vi "Get Indicator Number.vi"(8 "error in (no error)":errorcluster, 11 "Controls[]":refnum<vi>[](array[refnum])) -> (0 "error out":errorcluster, 3 "size(s)":i32)   [LabVIEW 2018, in "NISAST VI Scripting.lvlib" / "VI.lvlib" / "Front Panel.lvlib"]
uses:
  Front Panel.lvlib
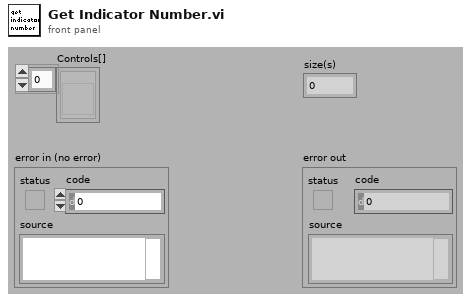
[diagram p1: front panel]
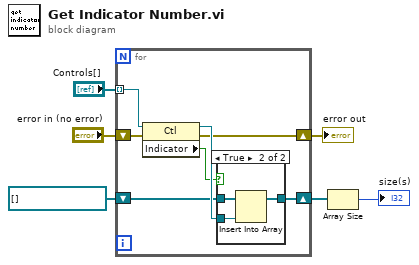
[diagram p0: block diagram]
diagram:
  n1 = for {
    tunnel: "Controls[]" -> [w13] mode=indexing
    shift-right: [w10] -> w4
    shift-left: refnum<vi>[] [] ("Controls[] 2") -> [w11]
    shift-right: [w7] -> w1
    shift-left: "error in (no error)" -> [w8]
    n2 = property class="Ctl"(reference=w13, error in=w8) -> (reference out=w12:refnum<vi>, error out=w7:errorcluster, "Indicator"=w9:bool)
    n3 = case shown="True" w9 {
      tunnel: w12 -> [_ w17]
      tunnel: w11 -> [w14 w16]
      tunnel: [w14 w15] -> w10
      frame False {
      }
      frame True {
        n4 = Insert Into Array(array=w16, new element=w17) -> (w15:refnum<vi>[])  [unwired: 1 in]
      }
    }
  }
  "error out" <- w1
  n5 = Array Size(array=w4) -> (size(s)=→"size(s)":i32)
